vi "Main aplication.vi"() -> ()   [LabVIEW 2020]
uses:
  Estados.ctl
  Cluster de informacion.ctl
  <vilib>/numeric/Random Number (Range) DBL.vi
  Variables Globales.vi
panel:
  out "Luz de Modo Manual":bool
  in  "Válvula Manual":dbl(knob) scale=0.0..1.0
  out "Lllenado completado":bool
  out "Flujo Volumétrico":dbl(graph)
  in  "Vaciar pote":bool
  out "LCD":string
  out "Apertura de la válvula":dbl(knob) scale=0.0..1.0
  out "Peso del pote de yogurt":dbl(slide) scale=0.0..1000.0
  in  "Tanque de yogurt":dbl(slide) scale=0.2..200.0
  in  "stop":bool
  in  "Suiche de pote de yogurt":bool
  out "Emergencia":bool
  out "Luz de Ajuste":bool
  in  "Modo Manual":bool
  in  "Parada de emergencia":bool
  in  "Activar-Desactivar\nModo ajuste":bool
  in  "Enter Tanque":bool
  in  "Cantidad de\nYogurt":dbl(knob) scale=0.0..900.0
  out "Nivel de \nTanque  Bajo":bool
  # "Pantalla LCD"
  # "Luces de Alerta"
  # "Panel de Control"
  # "Botones"
  # "Herramienas de Debbuging (No pertenece al sistema real)"
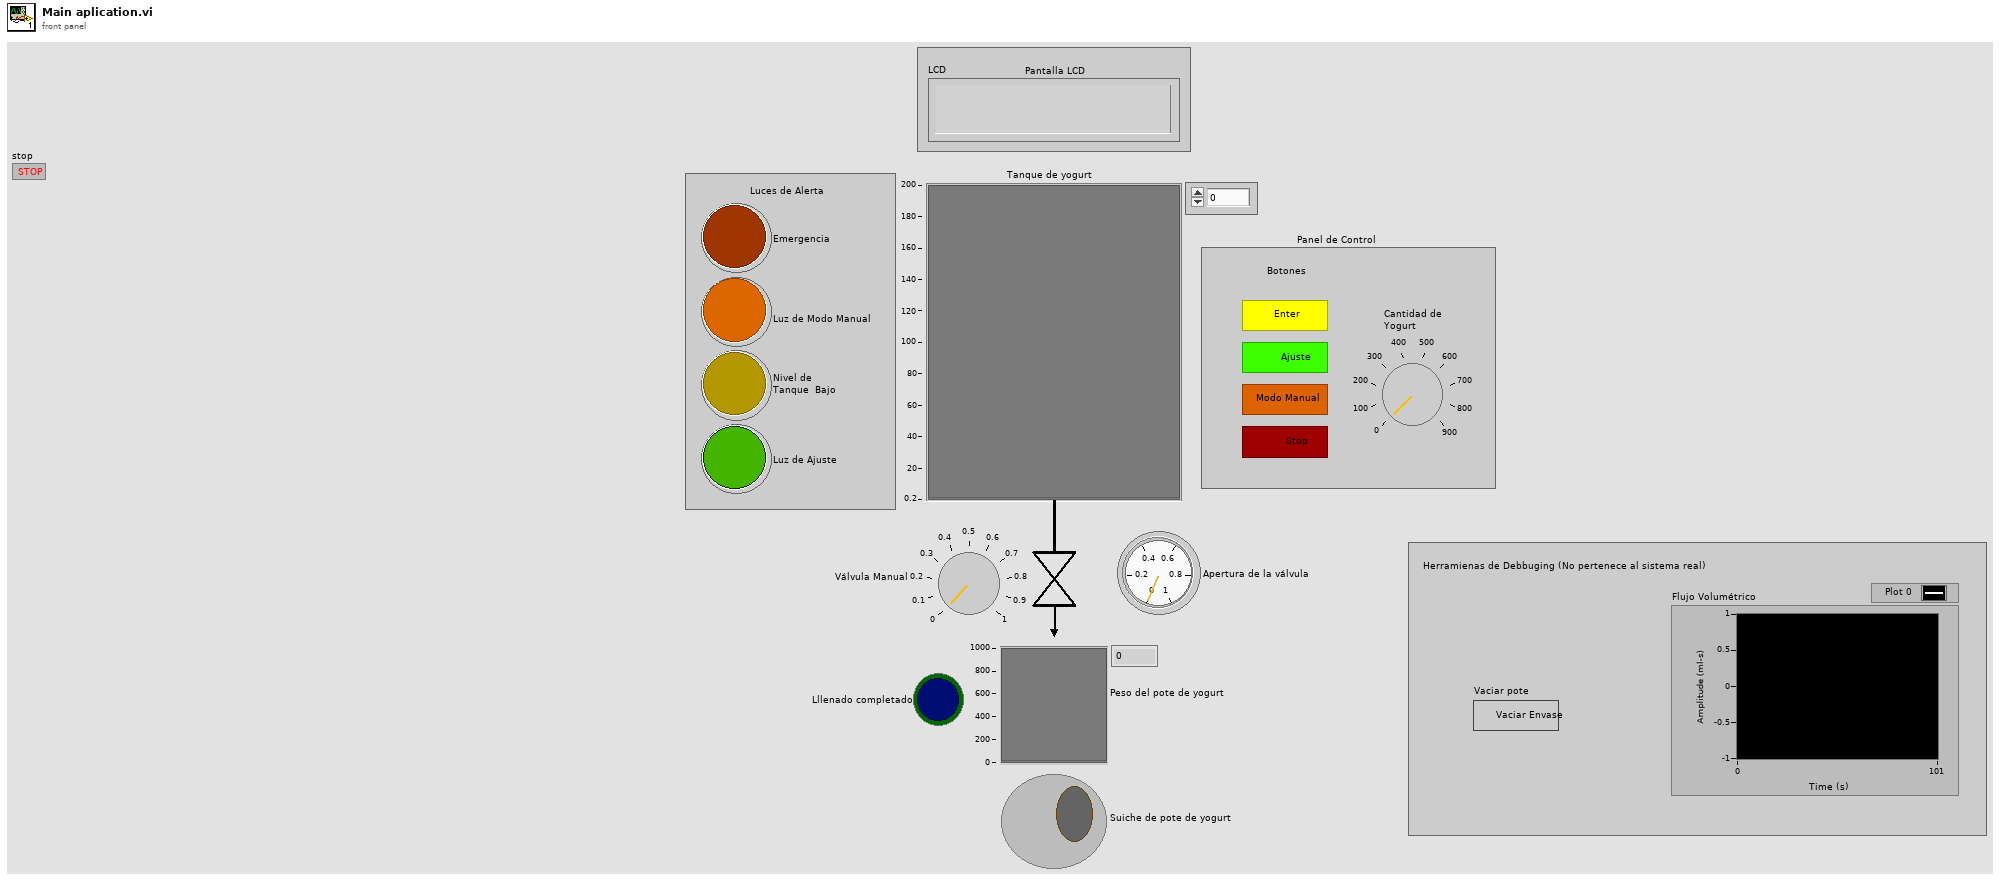
[diagram p1: front panel]
types:
  T1 = typedef "Cluster de informacion.ctl" = cluster{dbl, "Emergencia":bool, "Enter Tanque":bool, "Modo Ajuste":bool, "Error Msg":string}
  T2 = typedef "Estados.ctl" = enum16{"Errores?", "Modo Manual?", "Control de válvula alt.", "Control de válvula", "Nivel bajo?", "Query nivel del tanque", "Query peso del pote", "Ajuste?", "Llenado?", "Emergencia?", "Init", "Ajuste", "Nivel Bajo", "Llenado", "Error", "Emergencia"}
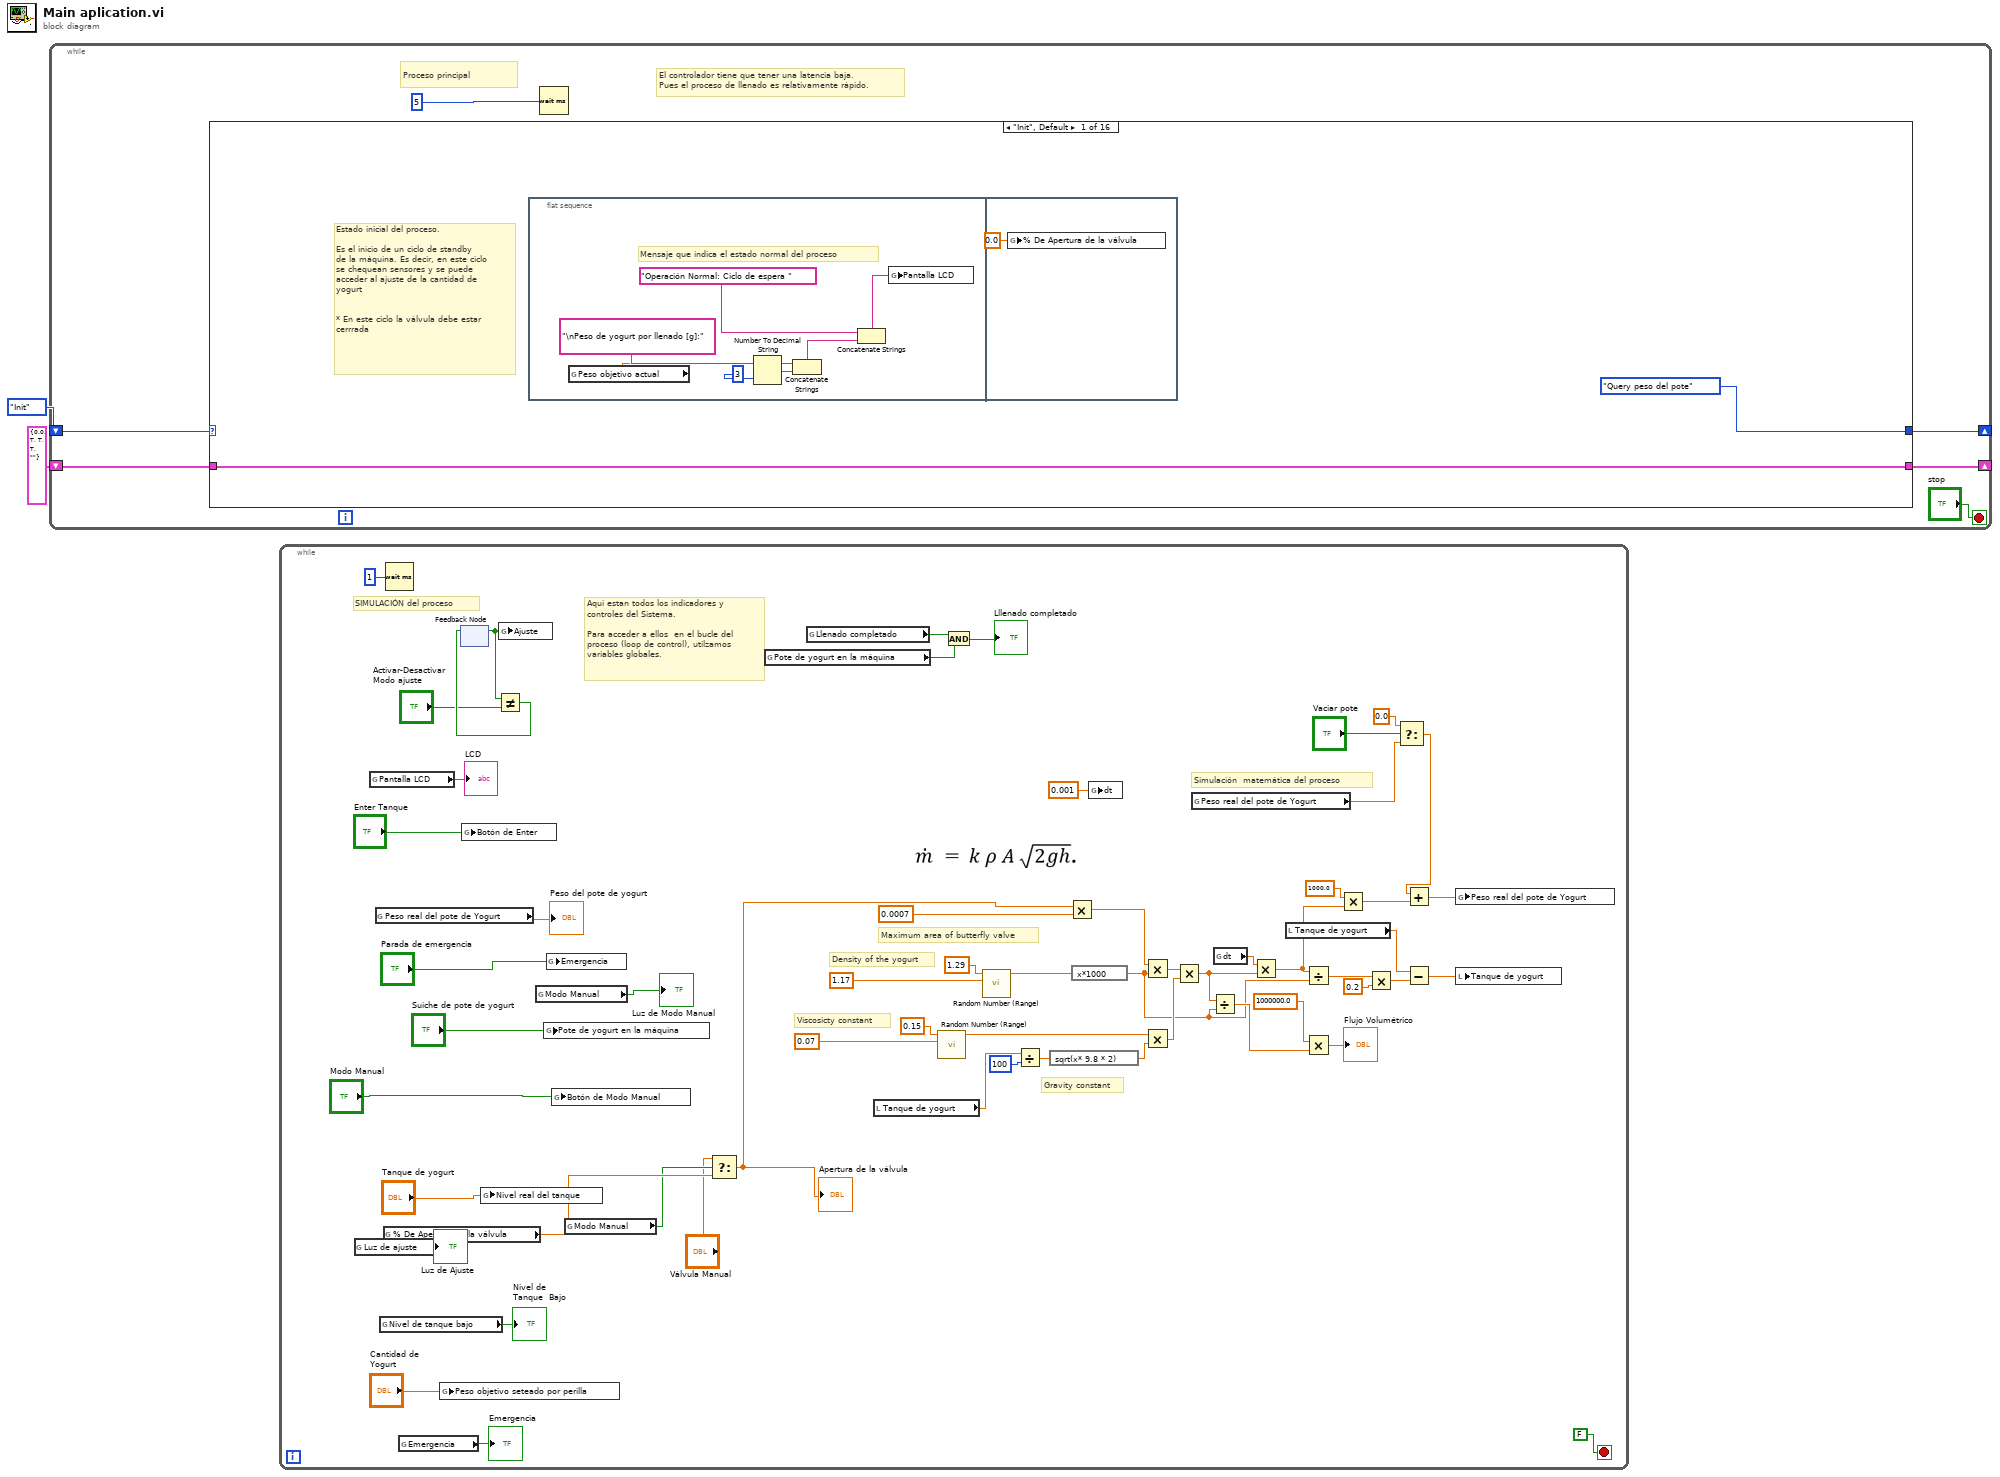
[diagram p0: block diagram]
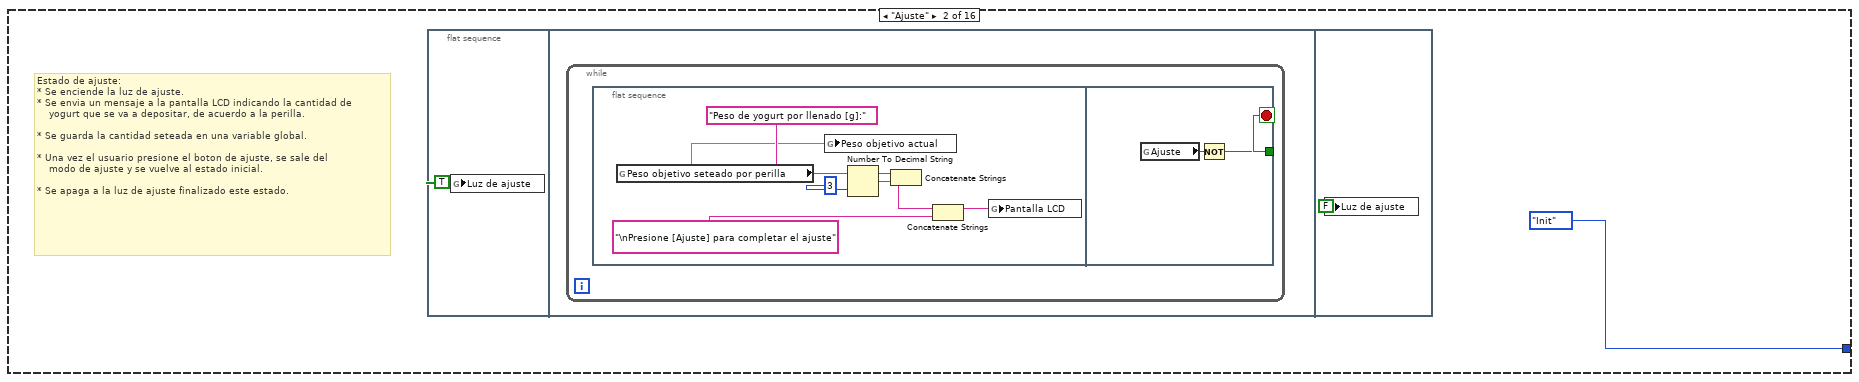
[diagram p2: hidden frame]
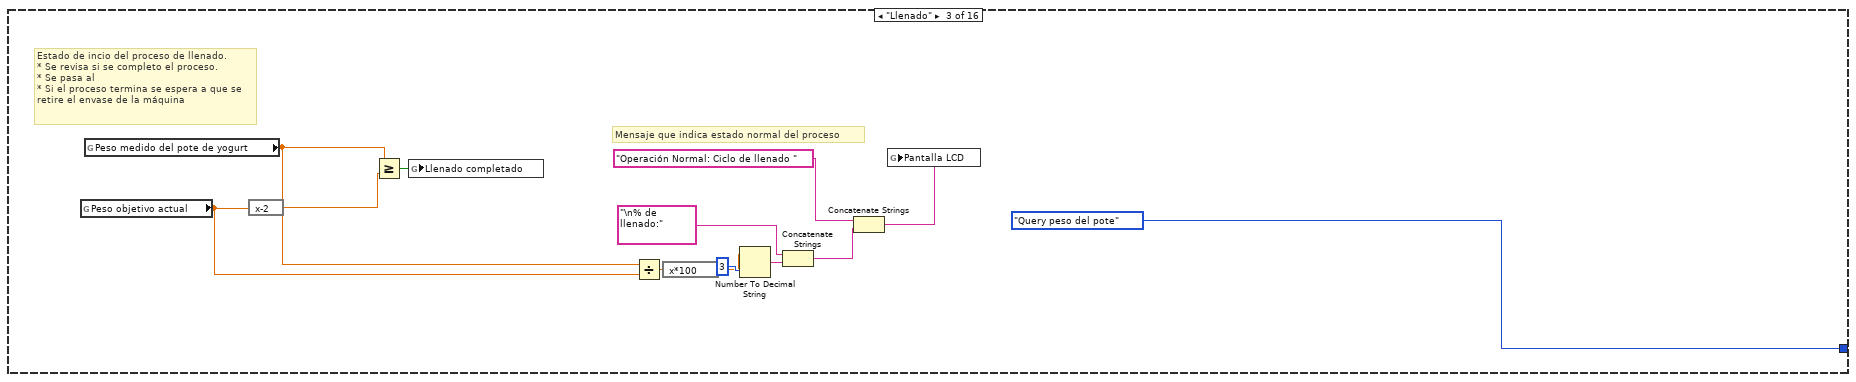
[diagram p3: hidden frame]
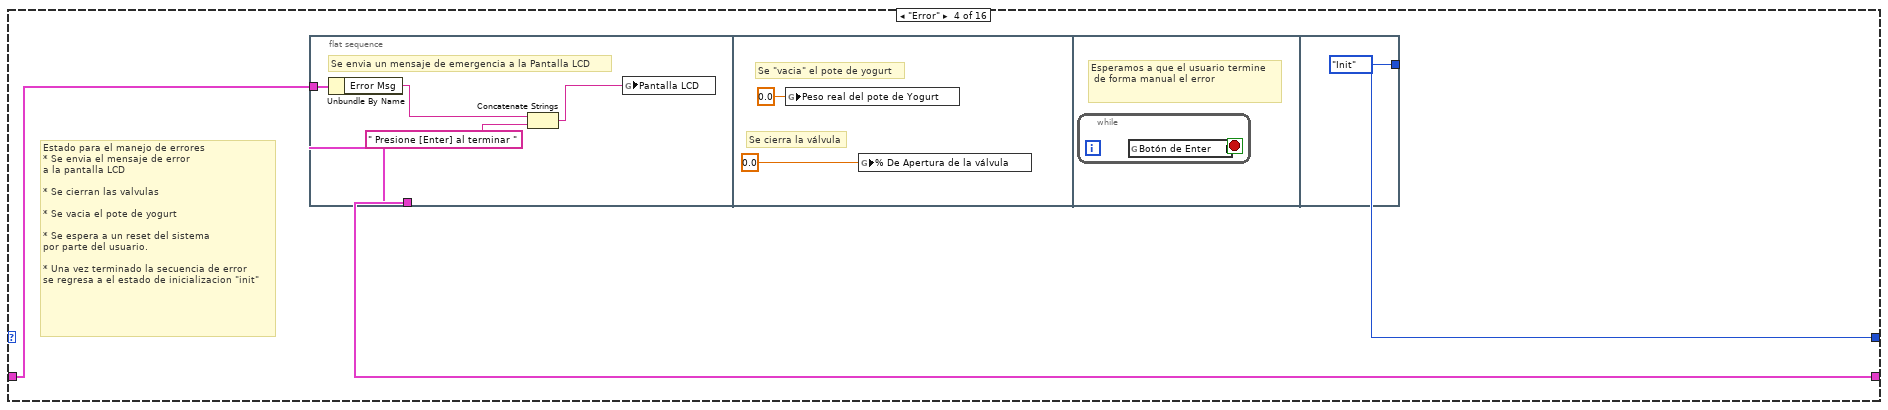
[diagram p4: hidden frame]
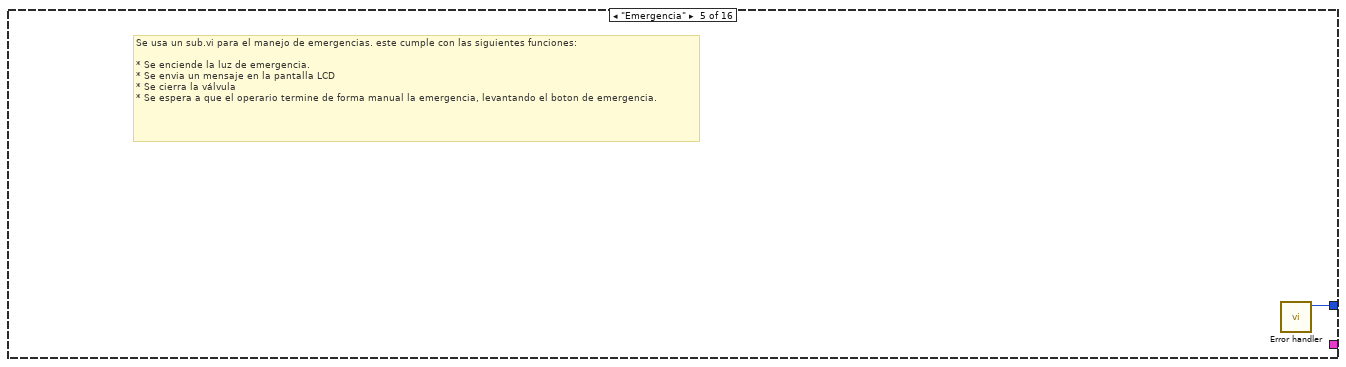
[diagram p5: hidden frame]
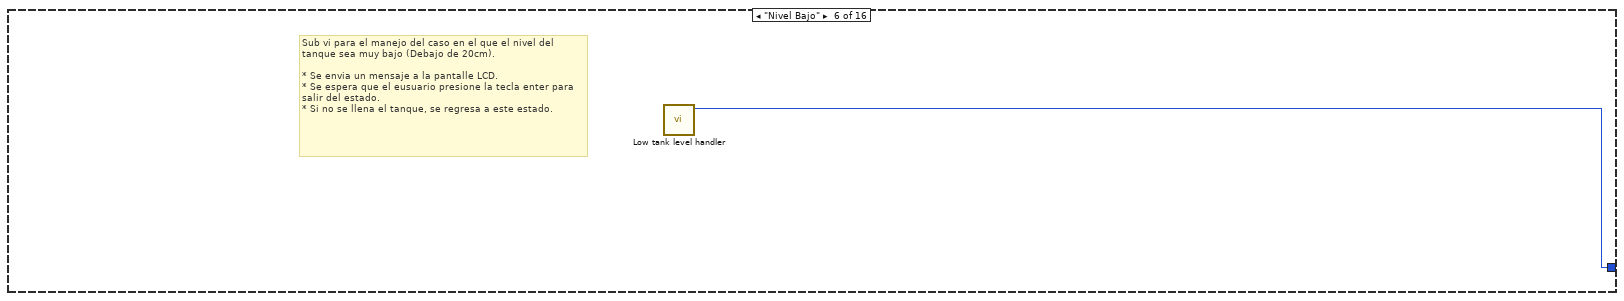
[diagram p6: hidden frame]
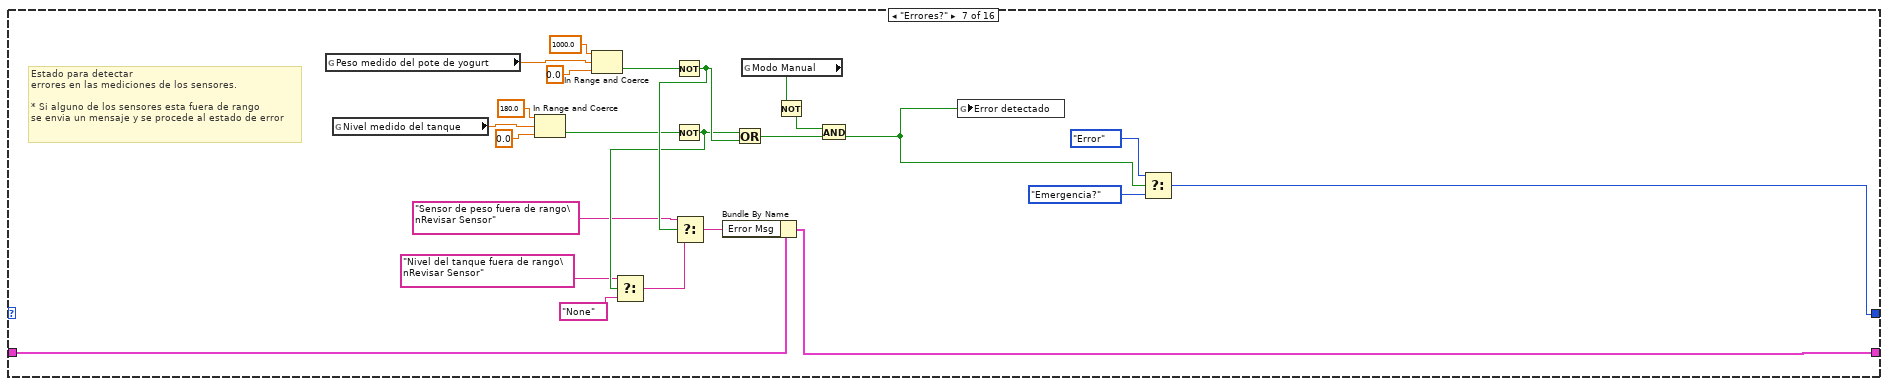
[diagram p7: hidden frame]
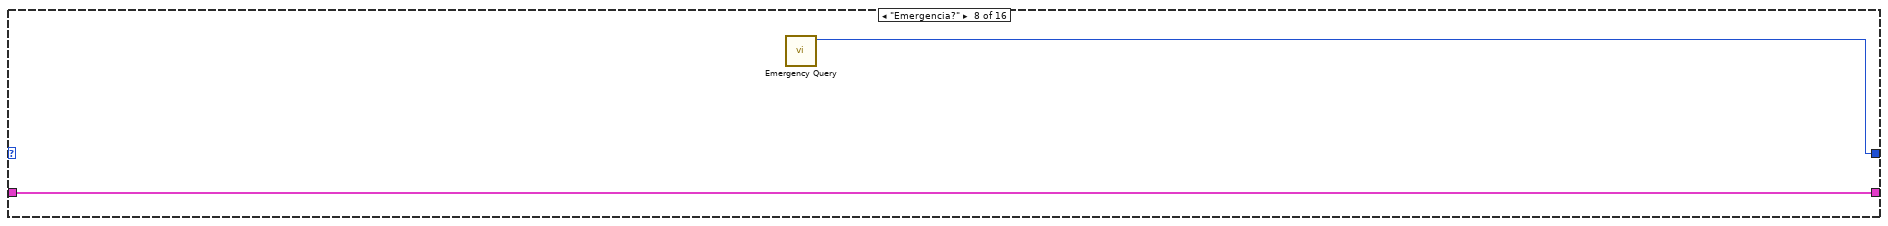
[diagram p8: hidden frame]
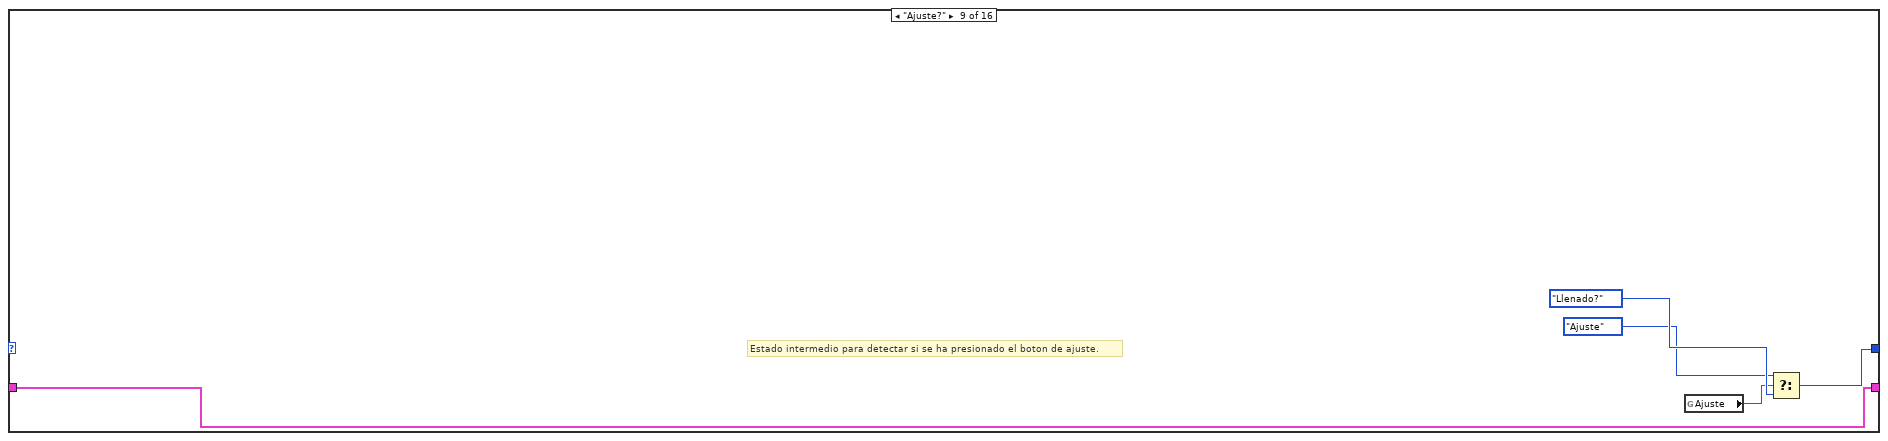
[diagram p9: hidden frame]
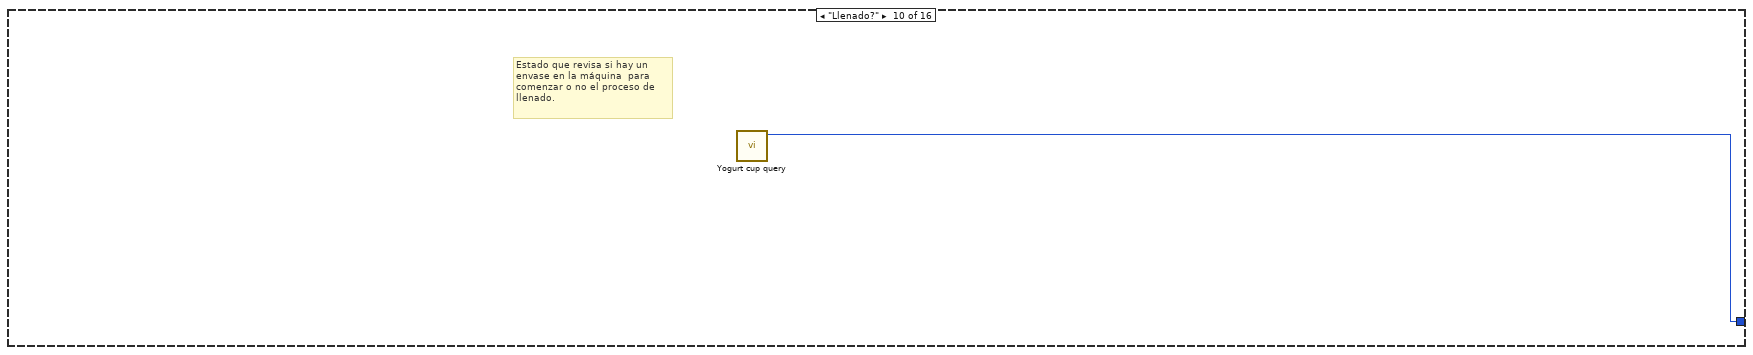
[diagram p10: hidden frame]
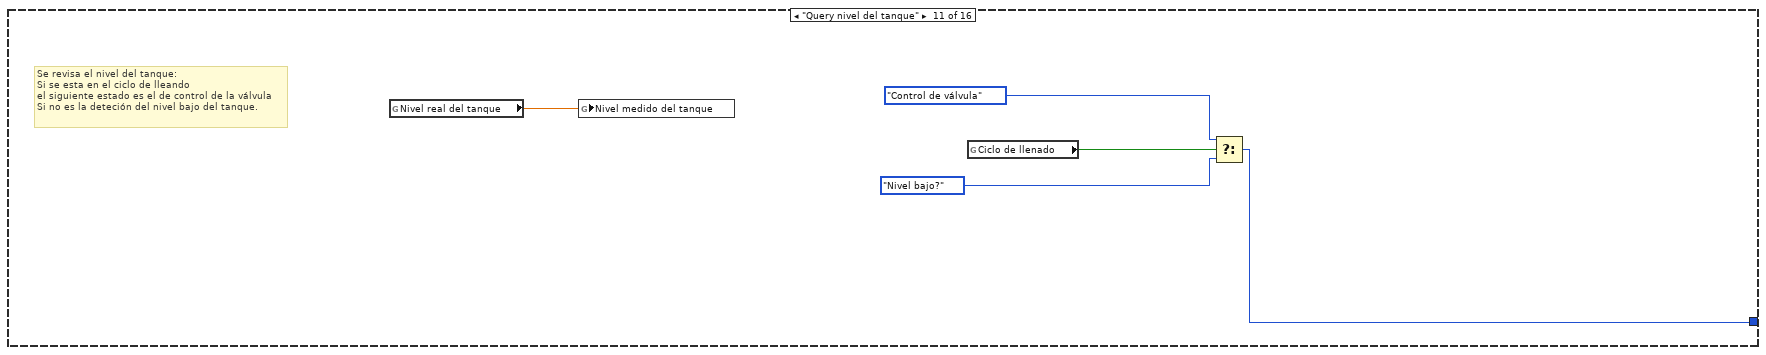
[diagram p11: hidden frame]
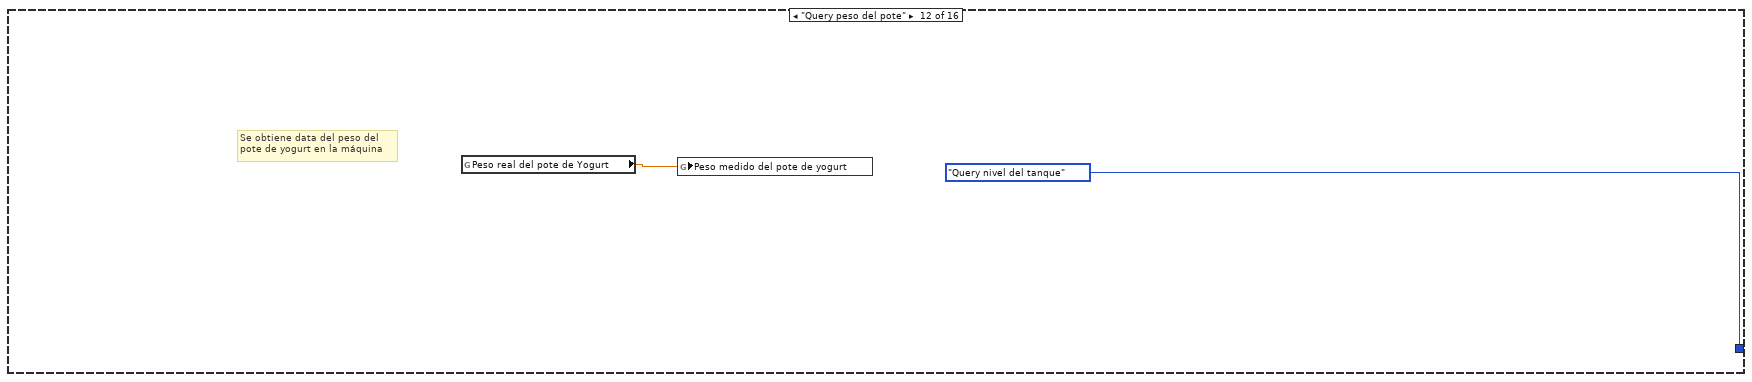
[diagram p12: hidden frame]
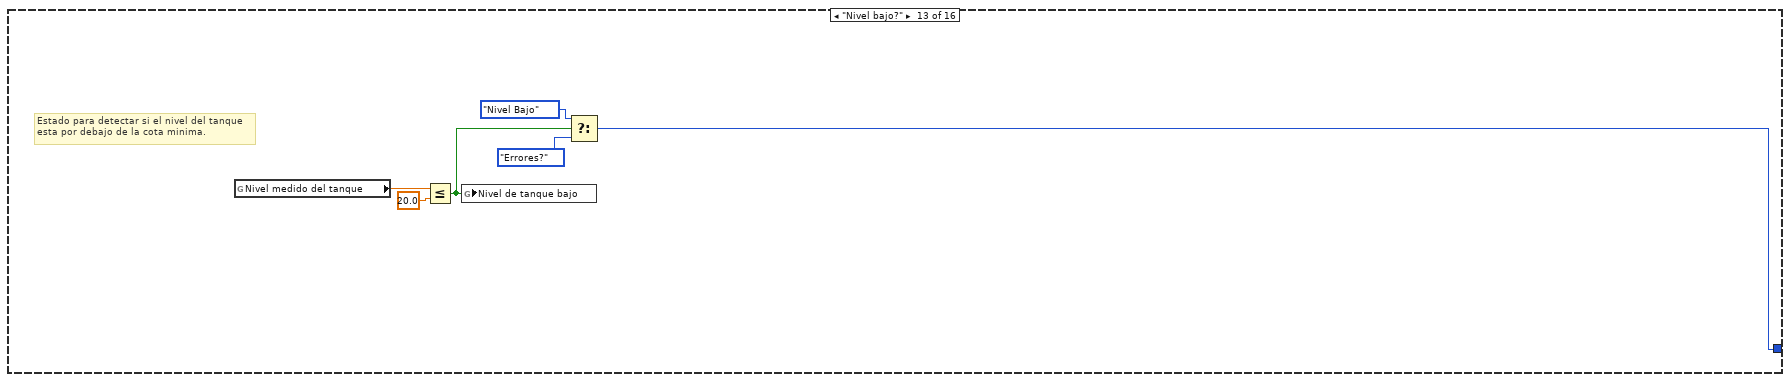
[diagram p13: hidden frame]
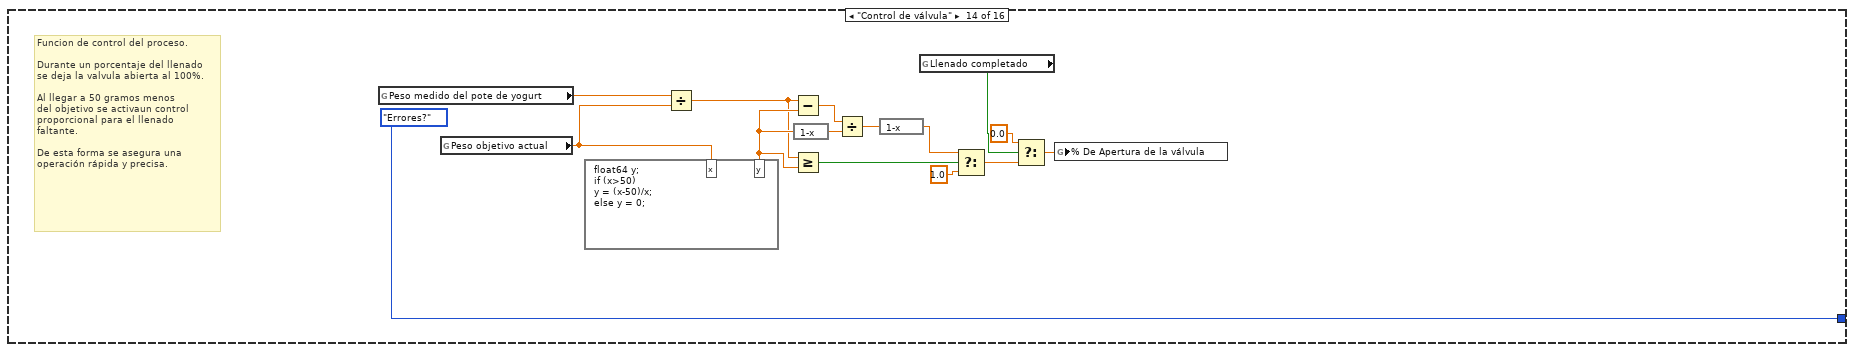
[diagram p14: hidden frame]
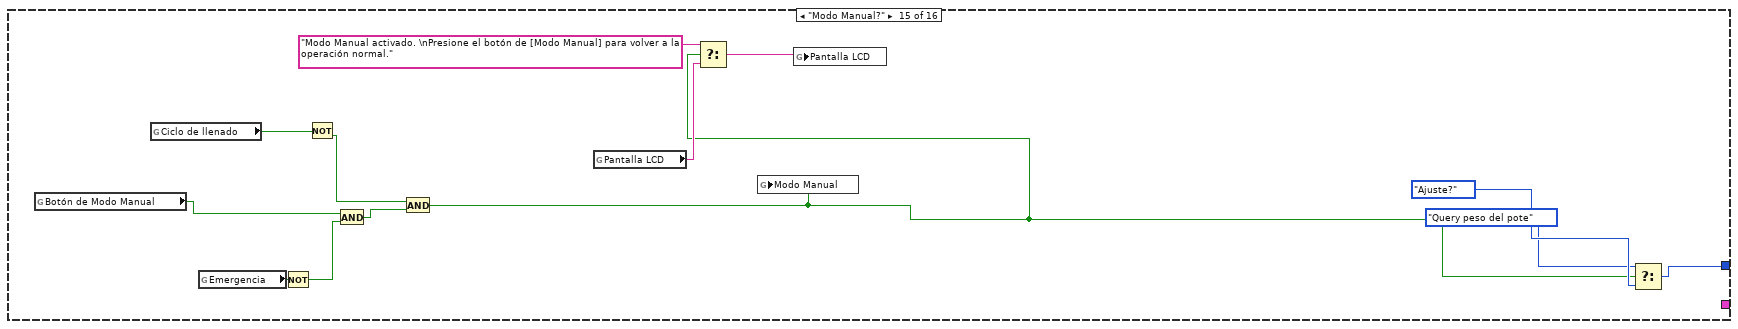
[diagram p15: hidden frame]
diagram:
  n1 = while {
    shift-right: [w7] -> _
    shift-left: Estados."Init" -> [w6]
    shift-right: [w3] -> _
    shift-left: T1 {0.0, "Emergencia"=TRUE, "Enter Tanque"=TRUE, "Modo Ajuste"=TRUE, "Error Msg"=""} -> [w4]
    stop <- "stop" stop-if-true
    # "El controlador tiene que tener una latencia baja.\nPues el proceso de llenado es relativamente rápido."
    # "Proceso principal"
    n2 = case shown="\"Init\", Default" w6 {
      tunnel: [Estados."Query peso del pote" Estados."Init" Estados."Query peso del pote" w45 w56 w57 w79 w83 w85 w89 w93 Estados."Query nivel del tanque" w98 Estados."Errores?" w128 _] -> w7
      tunnel: w4 -> [w9 _ _ w47 _ _ w70 w82 w84 _ _ _ _ _ _ _]
      tunnel: [w9 _ _ w46 _ _ w62 w82 w84 _ _ _ _ _ _ _] -> w3
      frame "Init", Default {
        # "Estado inicial del proceso.\n\nEs el inicio de un ciclo de standby\nde la máquina. Es decir, en este ciclo \nse chequean sensores y se puede \nacceder al ajuste de la cantidad de \nyogurt\n\n\n* En este ciclo la válvula debe estar \ncerrrada"
        n3 = flat-sequence {
          frame #0 {
            # "Mensaje que indica el estado normal del proceso"
            n4 = global read "Variables Globales.vi" "Peso objetivo actual"() -> (w14:dbl)
            n5 = Number To Decimal String(number=w14, width (-)=i16 3) -> (decimal integer string=w17:string)
            n6 = Concatenate Strings("\nPeso de yogurt por llenado [g]:" ("string"), w17) -> (w13:string)
            n7 = Concatenate Strings("Operación Normal: Ciclo de espera ", w13) -> (w11:string)
            n8 = global write "Variables Globales.vi" "Pantalla LCD"(w11) -> ()
          }
          frame #1 {
            n9 = global write "Variables Globales.vi" "% De Apertura de la válvula"(0.0 ("% De Apertura de la válvula")) -> ()
          }
        }
      }
      frame "Ajuste" {
        # "Estado de ajuste:\n* Se enciende la luz de ajuste.\n* Se envia un mensaje a la pantalla LCD indicando la cantidad de \n    yogurt que se va a depositar, de acuerdo a la perilla.\n\n* Se guarda la cantidad seteada en una variable global.\n\n* Una vez el usuario presione el boton de ajuste, se sale del \n    modo de ajuste y se vuelve al estado inicial.\n\n* Se apaga a la luz de ajuste finalizado este estado."
        n10 = flat-sequence {
          frame #0 {
            n11 = global write "Variables Globales.vi" "Luz de ajuste"(TRUE ("Luz de ajuste")) -> ()
          }
          frame #1 {
            n12 = while {
              stop <- w21 stop-if-true
              n13 = flat-sequence {
                tunnel: [w29] -> w21
                frame #0 {
                  n14 = global read "Variables Globales.vi" "Peso objetivo seteado por perilla"() -> (w25:dbl)
                  n15 = global write "Variables Globales.vi" "Peso objetivo actual"(w25) -> ()
                  n16 = Number To Decimal String(number=w25, width (-)=i16 3) -> (decimal integer string=w28:string)
                  n17 = Concatenate Strings("Peso de yogurt por llenado [g]:" ("string"), w28) -> (w23:string)
                  n18 = Concatenate Strings(w23, "\nPresione [Ajuste] para completar el ajuste") -> (w24:string)
                  n19 = global write "Variables Globales.vi" "Pantalla LCD"(w24) -> ()
                }
                frame #1 {
                  n20 = global read "Variables Globales.vi" "Ajuste"() -> (w30:bool)
                  n21 = Not(x=w30) -> (.not. x?=w29:bool)
                }
              }
            }
          }
          frame #2 {
            n22 = global write "Variables Globales.vi" "Luz de ajuste"(FALSE ("Luz de ajuste")) -> ()
          }
        }
      }
      frame "Llenado" {
        # "Mensaje que indica estado normal del proceso"
        # "Estado de incio del proceso de llenado.\n* Se revisa si se completo el proceso.\n* Se pasa al \n* Si el proceso termina se espera a que se \nretire el envase de la máquina"
        n23 = global read "Variables Globales.vi" "Peso objetivo actual"() -> (w35:dbl)
        n24 = global read "Variables Globales.vi" "Peso medido del pote de yogurt"() -> (w36:dbl)
        n25 = expression code="x-2"(w35) -> (w43:dbl)
        n26 = Greater Or Equal?(x=w36, y=w43) -> (x >= y?=w42:bool)
        n27 = global write "Variables Globales.vi" "Llenado completado"(w42) -> ()
        n28 = Divide(x=w36, y=w35) -> (x/y=w33:dbl)
        n29 = expression code="x*100"(w33) -> (w32:dbl)
        n30 = Number To Decimal String(number=w32, width (-)=i16 3) -> (decimal integer string=w39:string)
        n31 = Concatenate Strings("\n% de llenado:" ("string"), w39) -> (w40:string)
        n32 = Concatenate Strings("Operación Normal: Ciclo de llenado ", w40) -> (w41:string)
        n33 = global write "Variables Globales.vi" "Pantalla LCD"(w41) -> ()
      }
      frame "Error" {
        # "Estado para el manejo de errores\n* Se envia el mensaje de error\na la pantalla LCD\n\n* Se cierran las valvulas\n\n* Se vacia el pote de yogurt\n\n* Se espera a un reset del sistema\npor parte del usuario.\n\n* Una vez terminado la secuencia de error\nse regresa a el estado de inicializacion \"init\""
        n34 = flat-sequence {
          tunnel: w47 -> [w51]
          tunnel: [w51] -> w46
          tunnel: [Estados."Init"] -> w45
          frame #0 {
            # "Se envia un mensaje de emergencia a la Pantalla LCD"
            n35 = Unbundle By Name(w51) -> ("Error Msg"=w50:string)
            n36 = Concatenate Strings(w50, " Presione [Enter] al terminar " ("string")) -> (w49:string)
            n37 = global write "Variables Globales.vi" "Pantalla LCD"(w49) -> ()
          }
          frame #1 {
            # "Se \"vacia\" el pote de yogurt"
            # "Se cierra la válvula"
            n38 = global write "Variables Globales.vi" "Peso real del pote de Yogurt"(0.0) -> ()
            n39 = global write "Variables Globales.vi" "% De Apertura de la válvula"(0.0) -> ()
          }
          frame #2 {
            # "Esperamos a que el usuario termine\n de forma manual el error"
            n40 = while {
              stop <- w54 stop-if-true
              n41 = global read "Variables Globales.vi" "Botón de Enter"() -> (w54:bool)
            }
          }
          frame #3 {
          }
        }
      }
      frame "Emergencia" {
        # "Se usa un sub.vi para el manejo de emergencias. este cumple con las siguientes funciones:\n\n* Se enciende la luz de emergencia.\n* Se envia un mensaje en la pantalla LCD\n* Se cierra la válvula\n* Se espera a que el operario termine de forma manual la emergencia, levantando el boton de emergencia."
        n42 = call "Error handler.vi"() -> ("Enum"=w56:T2)  [unwired: 11 in]
      }
      frame "Nivel Bajo" {
        # "Sub vi para el manejo del caso en el que el nivel del\ntanque sea muy bajo (Debajo de 20cm).\n\n* Se envia un mensaje a la pantalle LCD.\n* Se espera que el eusuario presione la tecla enter para\nsalir del estado.\n* Si no se llena el tanque, se regresa a este estado."
        n43 = call "Low tank level handler.vi"() -> ("Enum"=w57:T2)  [unwired: 11 in]
      }
      frame "Errores?" {
        # "Estado para detectar\nerrores en las mediciones de los sensores.\n\n* Si alguno de los sensores esta fuera de rango\nse envia un mensaje y se procede al estado de error"
        n44 = global read "Variables Globales.vi" "Peso medido del pote de yogurt"() -> (w72:dbl)
        n45 = global read "Variables Globales.vi" "Nivel medido del tanque"() -> (w71:dbl)
        n46 = In Range and Coerce(upper limit=180.0, x=w71, lower limit=0.0) -> (In Range?=w74:bool)  [unwired: 1 out]
        n47 = In Range and Coerce(upper limit=1000.0, x=w72, lower limit=0.0) -> (In Range?=w75:bool)  [unwired: 1 out]
        n48 = Not(x=w75) -> (.not. x?=w78:bool)
        n49 = Not(x=w74) -> (.not. x?=w77:bool)
        n50 = Select(t="Nivel del tanque fuera de rango\nRevisar Sensor", s=w77, f="None") -> (s? t:f=w73:string)
        n51 = Select(t="Sensor de peso fuera de rango\nRevisar Sensor", s=w78, f=w73) -> (s? t:f=w76:string)
        n52 = Bundle By Name(cluster=w70, "Error Msg"=w76) -> (w62:T1)
        n53 = Or(x=w77, y=w78) -> (x .or. y?=w61:bool)
        n54 = global read "Variables Globales.vi" "Modo Manual"() -> (w59:bool)
        n55 = Not(x=w59) -> (.not. x?=w58:bool)
        n56 = And(x=w58, y=w61) -> (x .and. y?=w60:bool)
        n57 = global write "Variables Globales.vi" "Error detectado"(w60) -> ()
        n58 = Select(t=Estados."Error", s=w60, f=Estados."Emergencia?") -> (s? t:f=w79:T2)
      }
      frame "Emergencia?" {
        n59 = call "Emergency Query.vi"() -> ("Enum"=w83:T2)  [unwired: 11 in]
      }
      frame "Ajuste?" {
        # "Estado intermedio para detectar si se ha presionado el boton de ajuste."
        n60 = global read "Variables Globales.vi" "Ajuste"() -> (w86:bool)
        n61 = Select(t=Estados."Ajuste", s=w86, f=Estados."Llenado?") -> (s? t:f=w85:T2)
      }
      frame "Llenado?" {
        # "Estado que revisa si hay un \nenvase en la máquina  para \ncomenzar o no el proceso de \nllenado."
        n62 = call "Yogurt cup query.vi"() -> ("Enum"=w89:T2)  [unwired: 11 in]
      }
      frame "Query nivel del tanque" {
        # "Se revisa el nivel del tanque:\nSi se esta en el ciclo de lleando \nel siguiente estado es el de control de la válvula\nSi no es la deteción del nivel bajo del tanque."
        n63 = global read "Variables Globales.vi" "Nivel real del tanque"() -> (w94:dbl)
        n64 = global write "Variables Globales.vi" "Nivel medido del tanque"(w94) -> ()
        n65 = global read "Variables Globales.vi" "Ciclo de llenado"() -> (w92:bool)
        n66 = Select(t=Estados."Control de válvula", s=w92, f=Estados."Nivel bajo?") -> (s? t:f=w93:T2)
      }
      frame "Query peso del pote" {
        # "Se obtiene data del peso del\npote de yogurt en la máquina"
        n67 = global read "Variables Globales.vi" "Peso real del pote de Yogurt"() -> (w96:dbl)
        n68 = global write "Variables Globales.vi" "Peso medido del pote de yogurt"(w96) -> ()
      }
      frame "Nivel bajo?" {
        # "Estado para detectar si el nivel del tanque\nesta por debajo de la cota minima."
        n69 = global read "Variables Globales.vi" "Nivel medido del tanque"() -> (w102:dbl)
        n70 = Less Or Equal?(x=w102, y=20.0) -> (x <= y?=w97:bool)
        n71 = global write "Variables Globales.vi" "Nivel de tanque bajo"(w97) -> ()
        n72 = Select(t=Estados."Nivel Bajo", s=w97, f=Estados."Errores?") -> (s? t:f=w98:T2)
      }
      frame "Control de válvula" {
        # "Funcion de control del proceso.\n\nDurante un porcentaje del llenado \nse deja la valvula abierta al 100%.\n\nAl llegar a 50 gramos menos \ndel objetivo se activaun control \nproporcional para el llenado \nfaltante.\n\nDe esta forma se asegura una \noperación rápida y precisa."
        n73 = global read "Variables Globales.vi" "Peso medido del pote de yogurt"() -> (w109:dbl)
        n74 = global read "Variables Globales.vi" "Peso objetivo actual"() -> (w115:dbl)
        n75 = formula code="float64 y;\nif (x>50)\ny = (x-50)/x;\nelse y = 0;"("x"=w115) -> ("y"=w116:dbl)
        n76 = Divide(x=w109, y=w115) -> (x/y=w113:dbl)
        n77 = Subtract(x=w113, y=w116) -> (x-y=w110:dbl)
        n78 = Greater Or Equal?(x=w113, y=w116) -> (x >= y?=w107:bool)
        n79 = expression code="1-x"(w116) -> (w111:dbl)
        n80 = Divide(x=w110, y=w111) -> (x/y=w112:dbl)
        n81 = expression code="1-x"(w112) -> (w114:dbl)
        n82 = global read "Variables Globales.vi" "Llenado completado"() -> (w103:bool)
        n83 = Select(t=w114, s=w107, f=1.0) -> (s? t:f=w108:dbl)
        n84 = Select(t=0.0, s=w103, f=w108) -> (s? t:f=w106:dbl)
        n85 = global write "Variables Globales.vi" "% De Apertura de la válvula"(w106) -> ()
      }
      frame "Modo Manual?" {
        n86 = global read "Variables Globales.vi" "Botón de Modo Manual"() -> (w118:bool)
        n87 = global read "Variables Globales.vi" "Ciclo de llenado"() -> (w123:bool)
        n88 = global read "Variables Globales.vi" "Emergencia"() -> (w120:bool)
        n89 = Not(x=w120) -> (.not. x?=w121:bool)
        n90 = Not(x=w123) -> (.not. x?=w124:bool)
        n91 = And(x=w118, y=w121) -> (x .and. y?=w122:bool)
        n92 = And(x=w124, y=w122) -> (x .and. y?=w119:bool)
        n93 = global read "Variables Globales.vi" "Pantalla LCD"() -> (w127:string)
        n94 = Select(t="Modo Manual activado. \nPresione el botón de [Modo Manual] para volver a la operación normal.", s=w119, f=w127) -> (s? t:f=w125:string)
        n95 = global write "Variables Globales.vi" "Modo Manual"(w119) -> ()
        n96 = global write "Variables Globales.vi" "Pantalla LCD"(w125) -> ()
        n97 = Select(t=Estados."Query peso del pote", s=w119, f=Estados."Ajuste?") -> (s? t:f=w128:T2)
      }
      frame "Control de válvula alt." {
      }
    }
    n98 = Wait (ms)(milliseconds to wait=u32 5) -> ()  [unwired: 1 out]
  }
  n99 = while {
    stop <- FALSE stop-if-true
    # "Aqui estan todos los indicadores y\ncontroles del Sistema.\n\nPara acceder a ellos  en el bucle del\nproceso (loop de control), utilzamos \nvariables globales."
    # "Viscosicty constant"
    # "Simulación  matemática del proceso"
    # "Gravity constant"
    # "Density of the yogurt"
    # "Maximum area of butterfly valve"
    # "SIMULACIÓN del proceso"
    n100 = global read "Variables Globales.vi" "Luz de ajuste"() -> (→"Luz de Ajuste":bool)
    n101 = global read "Variables Globales.vi" "Pantalla LCD"() -> (→"LCD":string)
    n102 = global read "Variables Globales.vi" "Peso real del pote de Yogurt"() -> (→"Peso del pote de yogurt":dbl)
    n103 = global read "Variables Globales.vi" "Nivel de tanque bajo"() -> (→"Nivel de \nTanque  Bajo":bool)
    n104 = global read "Variables Globales.vi" "% De Apertura de la válvula"() -> (w139:dbl)
    n105 = Wait (ms)(milliseconds to wait=u32 1) -> ()  [unwired: 1 out]
    n106 = global read "Variables Globales.vi" "Emergencia"() -> (→"Emergencia":bool)
    n107 = global write "Variables Globales.vi" "Peso objetivo seteado por perilla"("Cantidad de\nYogurt") -> ()
    n108 = feedback #1() -> (w140:bool)  [unwired: 1 in]
    n109 = global write "Variables Globales.vi" "Botón de Enter"("Enter Tanque") -> ()
    n110 = global write "Variables Globales.vi" "Nivel real del tanque"("Tanque de yogurt") -> ()
    n111 = Not Equal?(x=w140, y="Activar-Desactivar\nModo ajuste") -> (x != y?=w182:bool)
    n112 = feedback-in #1(w182) -> ()
    n113 = global write "Variables Globales.vi" "Ajuste"(w140) -> ()
    n114 = global read "Variables Globales.vi" "Modo Manual"() -> (→"Luz de Modo Manual":bool)
    n115 = global write "Variables Globales.vi" "Pote de yogurt en la máquina"("Suiche de pote de yogurt") -> ()
    n116 = global write "Variables Globales.vi" "Emergencia"("Parada de emergencia") -> ()
    n117 = global write "Variables Globales.vi" "Botón de Modo Manual"("Modo Manual") -> ()
    n118 = global read "Variables Globales.vi" "Modo Manual"() -> (w138:bool)
    n119 = Select(t="Válvula Manual", s=w138, f=w139) -> (s? t:f=w136:dbl)
    "Apertura de la válvula" <- w136
    n120 = global read "Variables Globales.vi" "Pote de yogurt en la máquina"() -> (w141:bool)
    n121 = global read "Variables Globales.vi" "Llenado completado"() -> (w143:bool)
    n122 = local read "Tanque de yogurt"() -> (w162:dbl)
    n123 = call-poly <vilib>:"Random Number (Range).vi"("lower bound (0)"=0.07, "upper bound (100)"=0.15) -> ("number"=w144:dbl)  [unwired: 9 in]
    n124 = And(x=w143, y=w141) -> (x .and. y?=→"Lllenado completado":bool)
    n125 = call-poly <vilib>:"Random Number (Range).vi"("lower bound (0)"=1.17, "upper bound (100)"=1.29) -> ("number"=w157:dbl)  [unwired: 9 in]
    n126 = Divide(x=w162, y=u8 100) -> (x/y=w163:dbl)
    n127 = expression code="sqrt(x* 9.8 * 2)"(w163) -> (w171:dbl)
    n128 = Multiply(x=w136, y=0.0007) -> (x*y=w174:dbl)
    n129 = expression code="x*1000"(w157) -> (w149:dbl)
    n130 = global write "Variables Globales.vi" "dt"(0.001 ("dt")) -> ()
    n131 = Multiply(x=w174, y=w149) -> (x*y=w170:dbl)
    n132 = Multiply(x=w144, y=w171) -> (x*y=w152:dbl)
    n133 = Multiply(x=w170, y=w152) -> (x*y=w151:dbl)
    n134 = global read "Variables Globales.vi" "Peso real del pote de Yogurt"() -> (w134:dbl)
    n135 = Divide(x=w151, y=w149) -> (x/y=w150:dbl)
    n136 = global read "Variables Globales.vi" "dt"() -> (w169:dbl)
    n137 = Multiply(x=w169, y=w151) -> (x*y=w166:dbl)
    n138 = local read "Tanque de yogurt"() -> (w168:dbl)
    n139 = Divide(x=w166, y=w149) -> (x/y=w158:dbl)
    n140 = Multiply(x=1000000.0, y=w150) -> (x*y=→"Flujo Volumétrico":dbl)
    n141 = Multiply(x=1000.0, y=w166) -> (x*y=w160:dbl)
    n142 = Multiply(x=w158, y=0.2) -> (x*y=w156:dbl)
    n143 = Select(t=0.0, s="Vaciar pote", f=w134) -> (s? t:f=w133:dbl)
    n144 = Add(x=w133, y=w160) -> (x+y=w165:dbl)
    n145 = Subtract(x=w168, y=w156) -> (x-y=w167:dbl)
    n146 = global write "Variables Globales.vi" "Peso real del pote de Yogurt"(w165) -> ()
    n147 = local write "Tanque de yogurt"(w167) -> ()
  }
